vi "Update table.vi"(8 "error in":errorcluster, 10 "Seconds indicator":refnum<vi>, 11 "Table":refnum<vi>) -> (0 "error out":errorcluster)   [LabVIEW 2016]
uses:
  <vilib>/Utility/miscctls.llb/LVRowAndColumnTypeDef.ctl
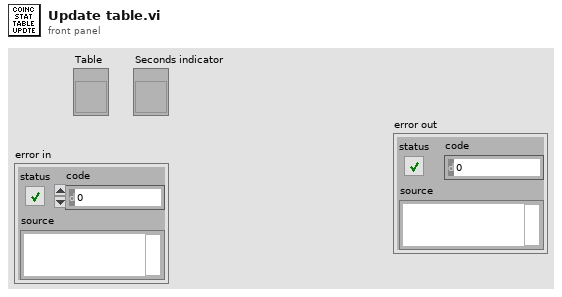
[diagram p1: front panel]
types:
  T1 = cluster{"Numofpoints":i32, "Current index":i32, "Max index":i32, "Data":cluster{"initialized array":i32[][], "Timestamp":timestamp}[], "Filled":bool}
  T2 = cluster{"initialized array":i32[][], "Timestamp":timestamp}[]
  T3 = cluster{"initialized array":i32[][], "Timestamp":timestamp}
  T4 = typedef "LVRowAndColumnTypeDef.ctl" = cluster{"Row":i32, "Column":i32}
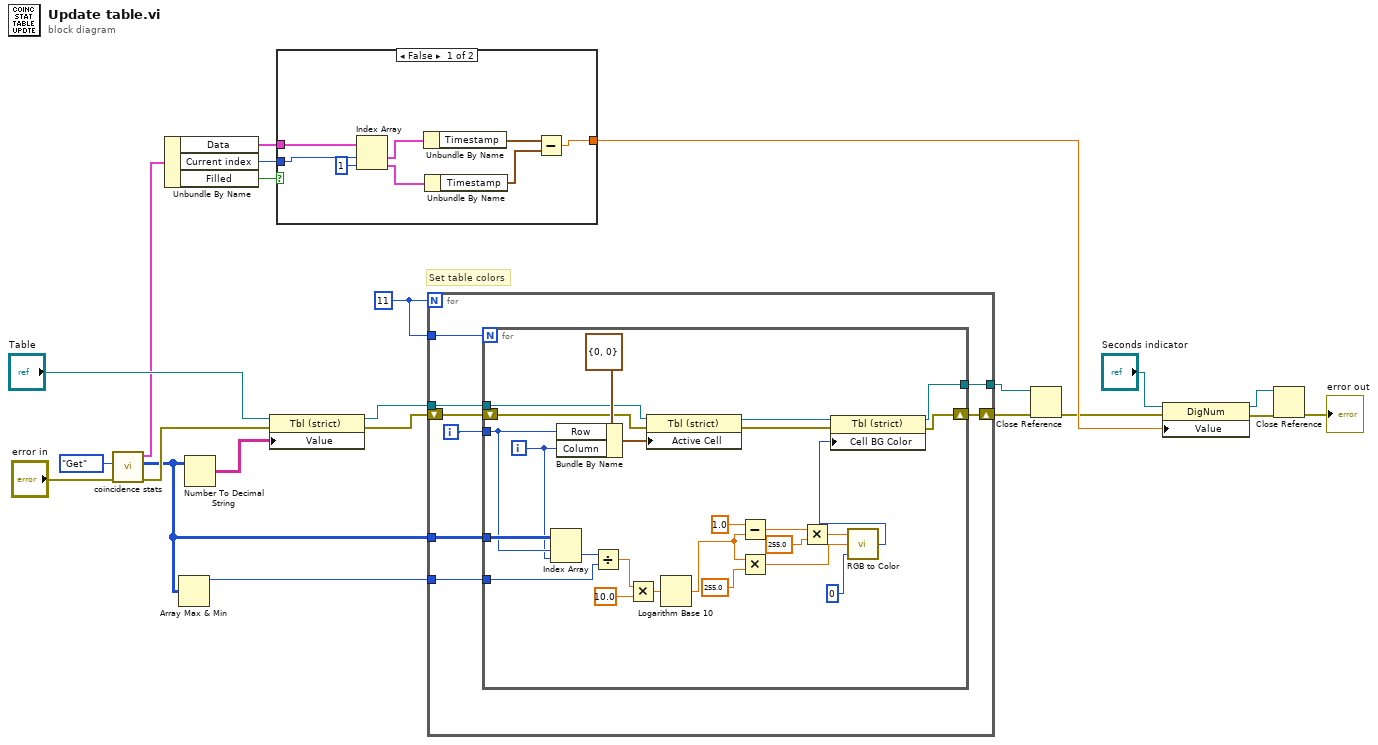
[diagram p0: block diagram]
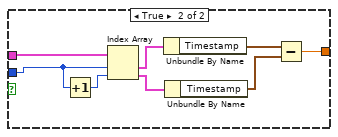
[diagram p2: hidden frame]
diagram:
  w11 = 11
  # "Set table colors"
  n1 = call "coincidence stats.vi"("error in"="error in", "Action"=enum16{"Insert", "Get", "Initiate"}."Get") -> ("error out"=w19:errorcluster, "Sum"=w17:i32[][], "Coinc stats"=w9:T1)  [unwired: 7 in]
  n2 = Unbundle By Name(w9) -> ("Data"=w7:T2, "Current index"=w8:i32, "Filled"=w10:bool)
  n3 = Array Max & Min(array=w17) -> (max value=w16:i32)  [unwired: 3 out]
  n4 = Number To Decimal String(number=w17) -> (decimal integer string=w20:string[][])  [unwired: 1 in]
  n5 = property class="Tbl (strict)"(reference="Table", error in=w19, "Value"=w20) -> (reference out=w14:refnum<vi>, error out=w15:errorcluster)
  n6 = case shown="False" w10 {
    tunnel: w8 -> [w29 w37]
    tunnel: w7 -> [w30 w38]
    tunnel: [w23 w31] -> w6
    frame False {
      n7 = Index Array(array=w30, index #1=w29, index #2=1 ("index")) -> (element #1=w25:T3, element #2=w24:T3)
      n8 = Unbundle By Name(w25) -> ("Timestamp"=w27:timestamp)
      n9 = Unbundle By Name(w24) -> ("Timestamp"=w26:timestamp)
      n10 = Subtract(x=w27, y=w26) -> (x-y=w23:dbl)
    }
    frame True {
      n11 = Increment(x=w37) -> (x+1=w36:i32)
      n12 = Index Array(array=w38, index #1=w37, index #2=w36) -> (element #1=w35:T3, element #2=w34:T3)
      n13 = Unbundle By Name(w35) -> ("Timestamp"=w33:timestamp)
      n14 = Unbundle By Name(w34) -> ("Timestamp"=w32:timestamp)
      n15 = Subtract(x=w33, y=w32) -> (x-y=w31:dbl)
    }
  }
  n16 = for {
    N: w11 -> [_]
    tunnel: w17 -> [w45]
    tunnel: w16 -> [w44]
    tunnel: w14 -> [w42]
    shift-right: [w41] -> w13
    shift-left: w15 -> [w43]
    tunnel: [w40] -> w12
    tunnel: w11 -> [w39]
    i -> [w46]
    n17 = for {
      N: w39 -> [_]
      tunnel: w46 -> [w68]
      tunnel: w45 -> [w69]
      tunnel: w44 -> [w65]
      tunnel: w42 -> [w53]
      shift-right: [w52] -> w41
      shift-left: w43 -> [w54]
      tunnel: [w51] -> w40
      i -> [w67]
      n18 = Index Array(array=w69, index (row)=w68, index (col)=w67) -> (element=w66:i32)
      n19 = Bundle By Name(cluster=T4 {"Row"=0, "Column"=0} ("Active Cell:Active Cell"), "Row"=w68, "Column"=w67) -> (w70:T4)
      n20 = Divide(x=w66, y=w65) -> (x/y=w50:dbl)
      n21 = Multiply(x=w50, y=10.0) -> (x*y=w48:dbl)
      n22 = property class="Tbl (strict)"(reference=w53, error in=w54, "Active Cell"=w70) -> (reference out=w55:refnum<vi>, error out=w57:errorcluster)
      n23 = Logarithm Base 10(1:w48) -> (0:w47:dbl)
      n24 = Subtract(x=1.0, y=w47) -> (x-y=w62:dbl)
      n25 = Multiply(x=w47, y=255.0) -> (x*y=w59:dbl)
      n26 = Multiply(x=w62, y=255.0) -> (x*y=w60:dbl)
      n27 = call <vilib>:"RGB to Color.vi"("B"=u8 0, "G"=w59, "R"=w60) -> ("Color"=w56:u32)
      n28 = property class="Tbl (strict)"(reference=w55, error in=w57, "Cell BG Color"=w56) -> (reference out=w51:refnum<vi>, error out=w52:errorcluster)
    }
  }
  n29 = Close Reference(reference=w12, error in (no error)=w13) -> (error out=w4:errorcluster)
  n30 = property class="DigNum"(reference="Seconds indicator", error in=w4, "Value"=w6) -> (reference out=w3:refnum<vi>, error out=w2:errorcluster)
  n31 = Close Reference(reference=w3, error in (no error)=w2) -> (error out=→"error out":errorcluster)
